vi "TranslatorBooster Translator.vi"() -> ()   [LabVIEW 2014, in "Complex Numbers.lvlib"]
uses:
  <vilib>/Aledyne-TSXperts/Arduino Compatible Compiler for LabVIEW/addons/Complex Numbers/Complex Numbers.lvlib
panel:
  out "Outputs":string[](array[string])
  out "Inputs":string[](array[string])
  out "Output Datatypes":string[](array[string])
  out "Input Datatypes":string[](array[string])
  out "Output":variant
  in  "Input":variant
  out "error out":errorcluster
  in  "error in (no error)":errorcluster
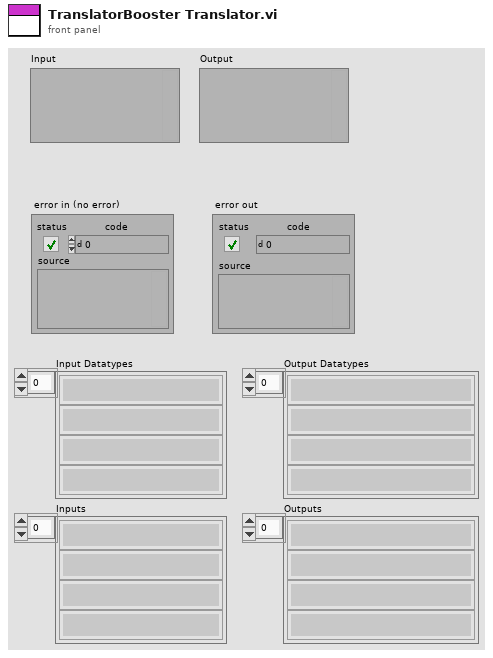
[diagram p1: front panel]
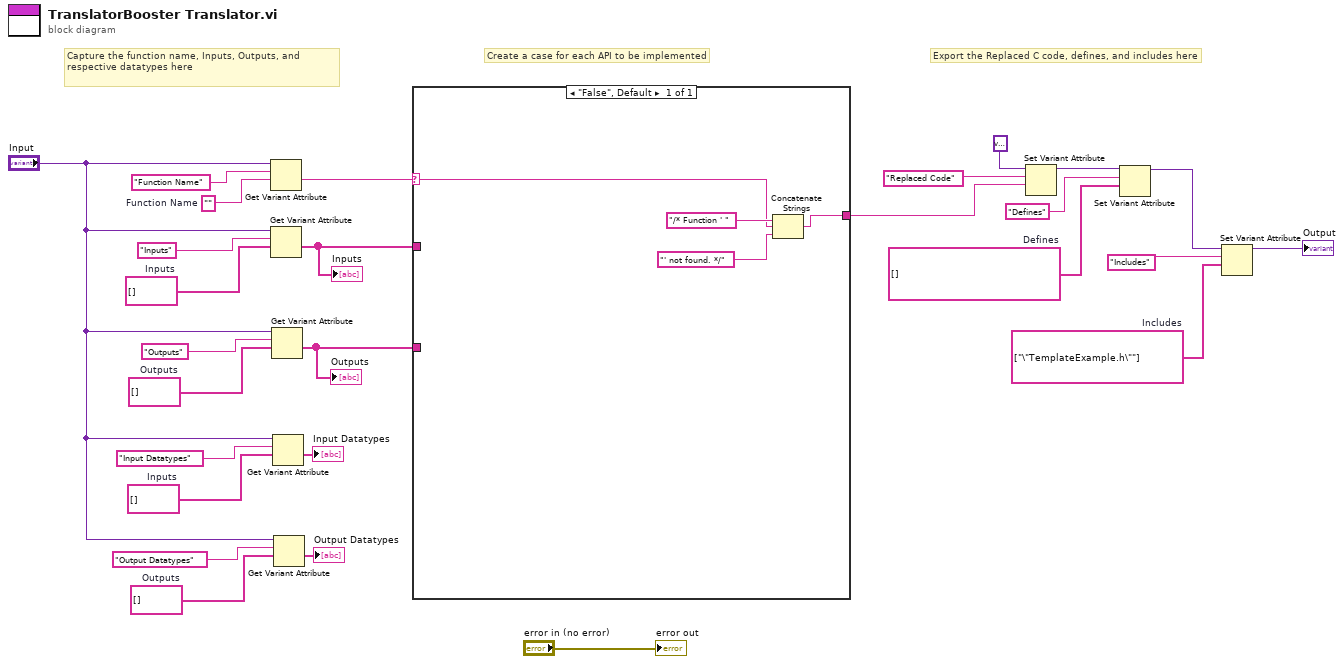
[diagram p0: block diagram]
diagram:
  w1 = string[] []  # Defines
  w12 = string[] []  # Outputs
  w13 = string[] []  # Inputs
  w18 = string[] ["\"TemplateExample.h\""]  # Includes
  w23 = string[] []  # Outputs
  w24 = string[] []  # Inputs
  w25 = ""  # Function Name
  # "Capture the function name, Inputs, Outputs, and respective datatypes here"
  # "Export the Replaced C code, defines, and includes here"
  # "Create a case for each API to be implemented"
  n1 = Get Variant Attribute(Variant="Input", name="Function Name", default value (empty Variant)=w25) -> (value=w20:string)  [unwired: 1 in, 3 out]
  n2 = Get Variant Attribute(Variant="Input", name="Inputs", default value (empty Variant)=w24) -> (value=w6:string[])  [unwired: 1 in, 3 out]
  "Inputs" <- w6
  n3 = Get Variant Attribute(Variant="Input", name="Outputs", default value (empty Variant)=w23) -> (value=w7:string[])  [unwired: 1 in, 3 out]
  "Outputs" <- w7
  n4 = Get Variant Attribute(Variant="Input", name="Input Datatypes", default value (empty Variant)=w13) -> (value=→"Input Datatypes":string[])  [unwired: 1 in, 3 out]
  n5 = Get Variant Attribute(Variant="Input", name="Output Datatypes", default value (empty Variant)=w12) -> (value=→"Output Datatypes":string[])  [unwired: 1 in, 3 out]
  n6 = case shown="\"False\", Default" w20 {
    selector: w20 -> [w29]
    tunnel: [w28] -> w19
    tunnel: w6 -> [_]
    tunnel: w7 -> [_]
    frame "False", Default {
      n7 = Concatenate Strings("/* Function ' ", w29, "' not found. */") -> (w28:string)
    }
  }
  n8 = Set Variant Attribute(Variant=variant ("variant"), name="Replaced Code", value=w19) -> (Variant out=w4:variant)  [unwired: 1 in, 2 out]
  n9 = Set Variant Attribute(Variant=w4, name="Defines", value=w1) -> (Variant out=w3:variant)  [unwired: 1 in, 2 out]
  n10 = Set Variant Attribute(Variant=w3, name="Includes", value=w18) -> (Variant out=→"Output":variant)  [unwired: 1 in, 2 out]
  "error out" <- "error in (no error)"
